vi "Kinesis - MST602 MNA601 - Two Axis Revector.vi"() -> ()   [LabVIEW 2012]
doc: "2D Revector example to centre a NanoTrak tracking power."
uses:
  U:/Kinesis LabVIEW Website Examples/Thorlabs.MotionControl.Controls.dll
  Thorlabs.MotionControl.Controls.dll
  U:/Kinesis LabVIEW Website Examples/Thorlabs.MotionControl.GenericMotorCLI.dll
  Thorlabs.MotionControl.GenericMotorCLI.dll
  U:/Kinesis LabVIEW Website Examples/Thorlabs.MotionControl.ModularRackCLI.dll
  Thorlabs.MotionControl.ModularRackCLI.dll
  U:/Kinesis LabVIEW Website Examples/Thorlabs.MotionControl.GenericNanoTrakCLI.dll
  Thorlabs.MotionControl.GenericNanoTrakCLI.dll
panel:
  out "Step Count":i32
  in  "Move (mm)":sgl=0.01
  in  "?":bool
  in  "?":bool
  in  "Revector Steps":i32=10
  in  "MNA601 SerialNumber":string
  in  "MST602 SerialNumber":string
  in  "ModularStepperControl -   Ch.1":refnum<k24>(container)
  in  "ModularStepperControl - Ch.2":refnum<k24>(container)
  in  "ModularNanoTrakControl":refnum<k24>(container)
  in  "Ch1":u32=4
  in  "Ch2":u32=4
  out "Error":errorcluster
  # "Thorlabs Hardware: \nMST602 Rack Module 2-Ch Stepper Motor Controller \nhttps://www.thorlabs.com/newgrouppage9.cfm?objectgroup_id=1186\n\nMNA601 Rack Module Fiber Auto-alignment Module\nhttps://www.thorlabs.com/newgrouppage9.cfm?objectgroup_id=1187\n\nDescription: The below VI will enable you to connect to a MNA601 & MST602.\nThe MNA601 provides users with an automated fibre alignment facility. It comprises of a PIN photodiode, Transimpedance Amplifier, & a dual channel High Voltage amplifier output circuit for driving two piezo actuators, typically found in our series of high precision flexure stages. The Nanotrak will drive the piezos via a PI servo loop, in a user adjustable circular motion to deduce the signal strength gradient for optimising & automating fibre alignment.\n\nAs the range of the Nanotrak operation is limited to the travel range of the piezo block, a revector routine will check the circle position & the MST602 is employed to control the connected motors, moving the circle position to centre. \n\nAn example of this application setup is pictured whereby the MST602 is driving will drive the internal X & Z piezo blocks of a MAX381 stage. The MAX381 stage is holding an optical fibre aligned to a waveguide in series with secondary receiving fibre via use of Thorlabs flexure stage holder accessories. The secondary fibre is mounted to a secondary co-located MAX302 stage. This fibre is connected to the Optical Input of the MNA601 controller.\n\nThe VI will stop once the revector routine is complete or the user has click 'END'. The user is able to set the number of Revector Iterations (Steps), as well as the step size of the motor movements as well as monitor the current step count.\n\nInstructions: \n1) Connect a MNA601 & MST602 to MMR601 as per the respective product user manuals. These can be connected to any bay in the MMR601 rack.\n2) Enter the module serial numbers below.\n3) Enter the Revector parameters (Move & Revector Iteration Count),\n4) To run the VI, click the run button in the LabVIEW Toolbar.\n5) Once running, the Kinesis UIs will initialise & the VI will wait for you to assign the correct motor types. This can be done by selecting the actuator type on the Kinesis device name on the UI panel & then click 'ACTUATOR SELECTED'\n4) The VI will exit when the revector iteration count is complete or 'END' is clicked."
  # "Notes:"
  # "- Ensure that the appropriate .DLLs are copied into your Project Folder. Check that the correct bit type are used depending on your version of LabVIEW\ni.e. 32-bit or 64-bit.\n\n\n\n\n\n\n\n\n\n\n\n\n\n\n- Open the example VI through the LabVIEW Project Explorer to correctly load the User Interface from Thorlabs.MotionControl.Controls.dll."
  # "Example Image of .NET Controller - VI opened via Project Explorer/ not opened via Project Explorer"
  # "VI Not Opened via Project Explorer"
  # "VI Opened via Project Explorer"
  # "- To explore the range of methods available, please visit the .NET API, included with your Kinesis software.\n\n- For tips on building your own VIs with Thorlabs Motion Control Hardware, please see our LabVIEW Guide here.\nhttps://www.thorlabs.com/newgrouppage9.cfm?objectgroup_id=10285"
  # "Motor Start Position\n(mm)"
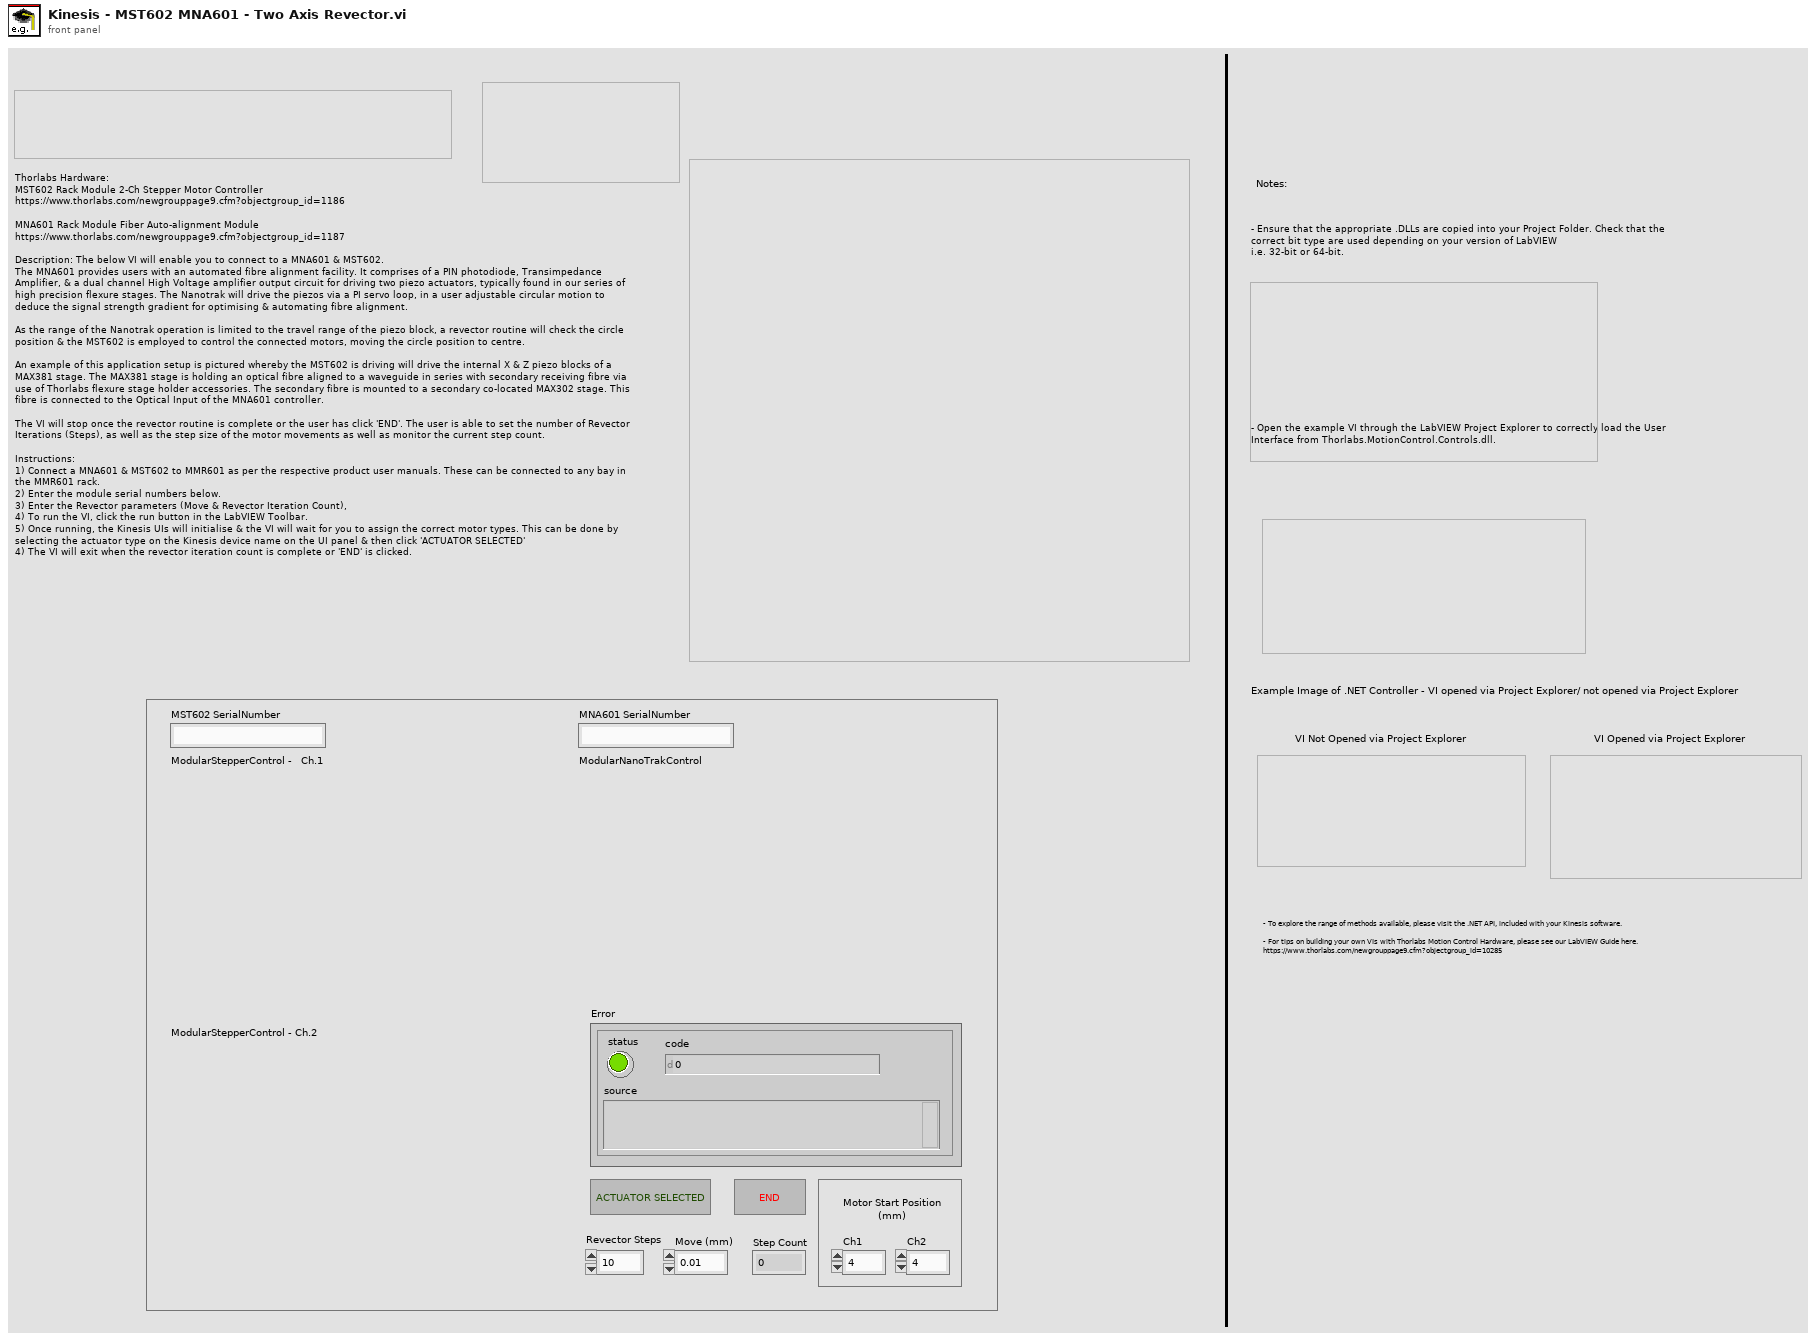
[diagram p1: front panel]
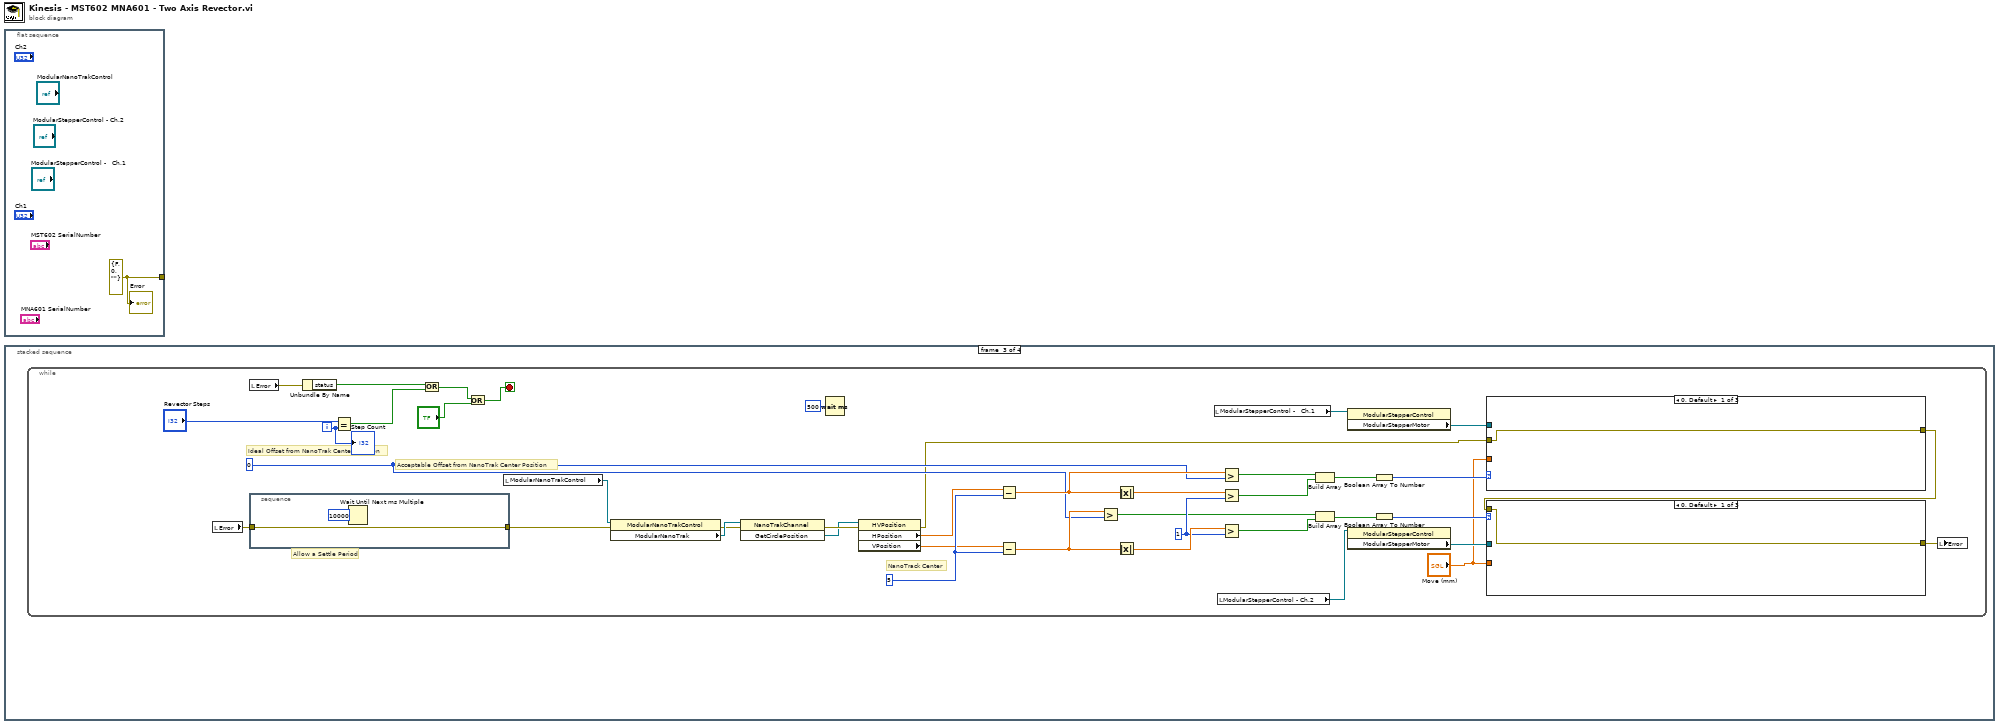
[diagram p0: block diagram]
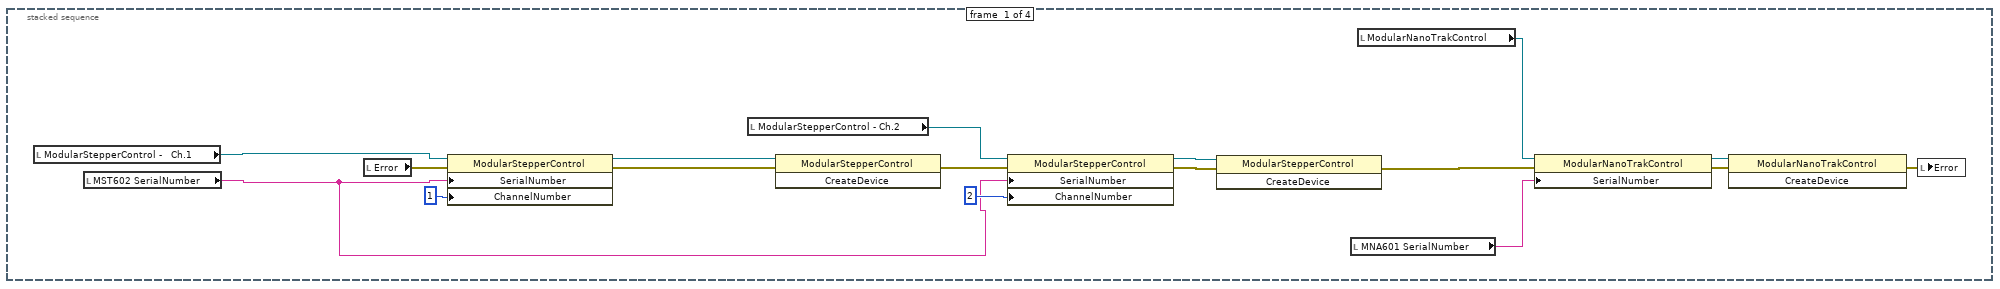
[diagram p2: hidden frame]
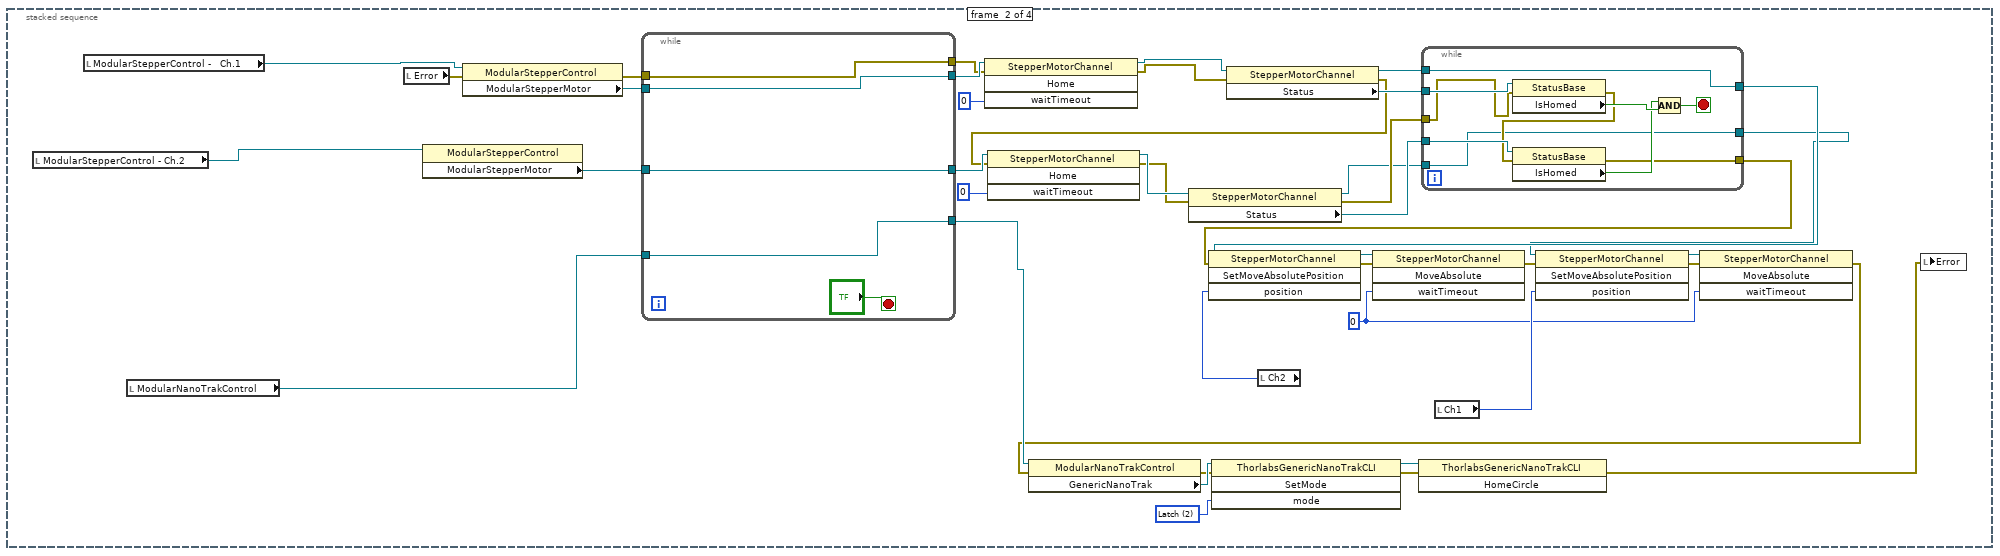
[diagram p3: hidden frame]
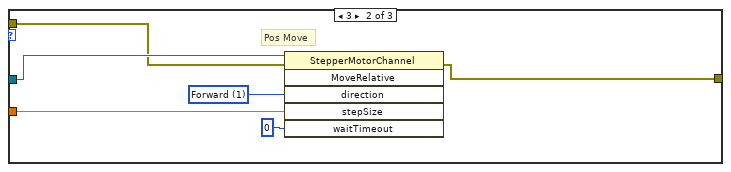
[diagram p4: hidden frame]
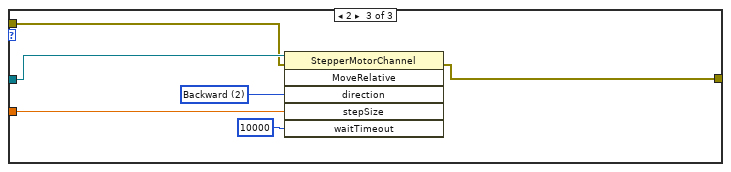
[diagram p5: hidden frame]
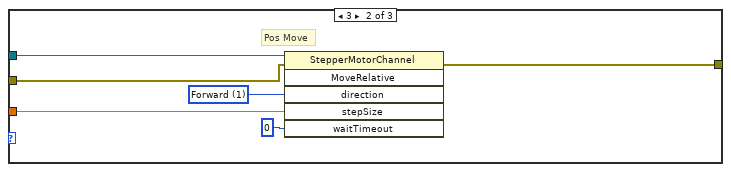
[diagram p6: hidden frame]
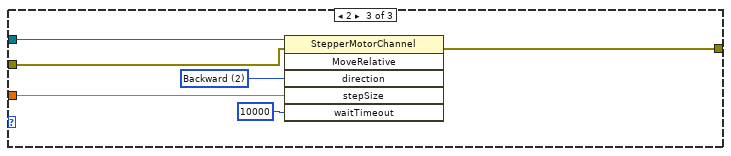
[diagram p7: hidden frame]
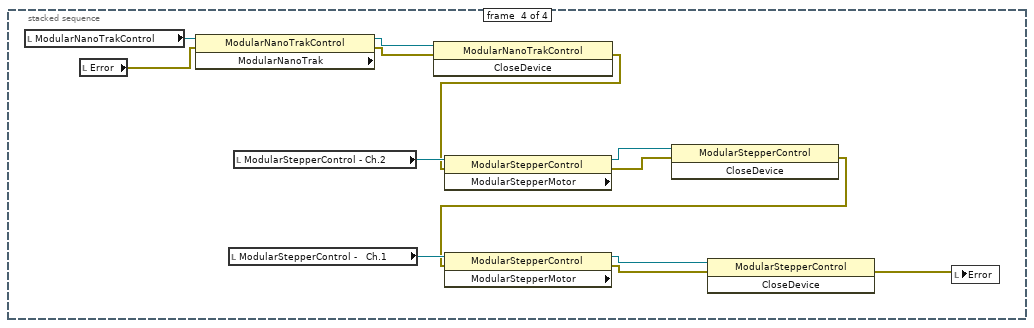
[diagram p8: hidden frame]
diagram:
  n1 = flat-sequence {
    tunnel: [w1] -> _
    frame #0 {
      w1 = errorcluster {"status"=FALSE, "code"=0, "source"=""} ("error in (no error)")
      "Error" <- w1
    }
  }
  n2 = stacked-sequence {
    frame #0 {
      n3 = local read "ModularStepperControl -   Ch.1"() -> (w7:refnum<k24>)
      n4 = local read "MST602 SerialNumber"() -> (w2:string)
      n5 = local read "Error"() -> (w16:errorcluster)
      n6 = property class="ModularStepperControl"(reference=w7, error in=w16, "SerialNumber"=w2, "ChannelNumber"=1) -> (reference out=w18:refnum<k24>, error out=w17:errorcluster)
      n7 = local read "ModularStepperControl - Ch.2"() -> (w3:refnum<k24>)
      n8 = invoke class="ModularStepperControl" method="CreateDevice"(reference=w18, error in=w17) -> (error out=w5:errorcluster)  [unwired: 1 in, 2 out]
      n9 = property class="ModularStepperControl"(reference=w3, error in=w5, "SerialNumber"=w2, "ChannelNumber"=2) -> (reference out=w9:refnum<k24>, error out=w15:errorcluster)
      n10 = invoke class="ModularStepperControl" method="CreateDevice"(reference=w9, error in=w15) -> (error out=w4:errorcluster)  [unwired: 1 in, 2 out]
      n11 = local read "MNA601 SerialNumber"() -> (w12:string)
      n12 = local read "ModularNanoTrakControl"() -> (w13:refnum<k24>)
      n13 = property class="ModularNanoTrakControl"(reference=w13, error in=w4, "SerialNumber"=w12) -> (reference out=w11:refnum<k24>, error out=w10:errorcluster)
      n14 = invoke class="ModularNanoTrakControl" method="CreateDevice"(reference=w11, error in=w10) -> (error out=w8:errorcluster)  [unwired: 1 in, 2 out]
      n15 = local write "Error"(w8) -> ()
    }
    frame #1 {
      w23 = 2 items=["Undefined", "Piezo", "Latch", "Tracking", "HorizontalTracking", "VerticalTracking"] ("mode")
      w48 = 0 ("waitTimeout")
      n16 = local read "ModularStepperControl - Ch.2"() -> (w57:refnum<k24>)
      n17 = local read "ModularStepperControl -   Ch.1"() -> (w58:refnum<k24>)
      n18 = local read "ModularNanoTrakControl"() -> (w21:refnum<k24>)
      n19 = local read "Error"() -> (w56:errorcluster)
      n20 = property class="ModularStepperControl"(reference=w57) -> ("ModularStepperMotor"=w43:refnum<k24>)  [unwired: 1 in, 2 out]
      n21 = property class="ModularStepperControl"(reference=w58, error in=w56) -> (error out=w41:errorcluster, "ModularStepperMotor"=w45:refnum<k24>)  [unwired: 1 out]
      n22 = while {
        tunnel: [w64] -> w46
        tunnel: w45 -> [w64]
        tunnel: [w63] -> w44
        tunnel: w43 -> [w63]
        tunnel: [w62] -> w42
        tunnel: w41 -> [w62]
        tunnel: [w60] -> w22
        tunnel: w21 -> [w60]
        stop <- "?" stop-if-true
      }
      n23 = invoke class="StepperMotorChannel" method="Home"(reference=w46, error in=w42, "waitTimeout"=0) -> (reference out=w37:refnum<k24>, error out=w40:errorcluster)  [unwired: 1 in, 2 out]
      n24 = property class="StepperMotorChannel"(reference=w37, error in=w40) -> (reference out=w30:refnum<k24>, error out=w35:errorcluster, "Status"=w38:refnum<k24>)
      n25 = invoke class="StepperMotorChannel" method="Home"(reference=w44, error in=w35, "waitTimeout"=0) -> (reference out=w36:refnum<k24>, error out=w34:errorcluster)  [unwired: 1 in, 2 out]
      n26 = property class="StepperMotorChannel"(reference=w36, error in=w34) -> (reference out=w28:refnum<k24>, error out=w33:errorcluster, "Status"=w39:refnum<k24>)
      n27 = local read "Ch2"() -> (w54:u32)
      n28 = while {
        tunnel: w39 -> [w71]
        tunnel: w38 -> [w70]
        tunnel: w33 -> [w68]
        tunnel: [w67] -> w32
        tunnel: [w66] -> w31
        tunnel: w30 -> [w66]
        tunnel: [w65] -> w29
        tunnel: w28 -> [w65]
        stop <- w72 stop-if-true
        n29 = property class="StatusBase"(reference=w70, error in=w68) -> (error out=w69:errorcluster, "IsHomed"=w74:bool)  [unwired: 1 out]
        n30 = property class="StatusBase"(reference=w71, error in=w69) -> (error out=w67:errorcluster, "IsHomed"=w73:bool)  [unwired: 1 out]
        n31 = Compound Arithmetic op=AND(w73, w74) -> (w72:bool)
      }
      n32 = invoke class="StepperMotorChannel" method="SetMoveAbsolutePosition"(reference=w31, error in=w32, "position"=w54) -> (reference out=w51:refnum<k24>, error out=w50:errorcluster)  [unwired: 1 in, 2 out]
      n33 = invoke class="StepperMotorChannel" method="MoveAbsolute"(reference=w51, error in=w50, "waitTimeout"=w48) -> (error out=w55:errorcluster)  [unwired: 1 in, 3 out]
      n34 = local read "Ch1"() -> (w53:u32)
      n35 = invoke class="StepperMotorChannel" method="SetMoveAbsolutePosition"(reference=w29, error in=w55, "position"=w53) -> (reference out=w52:refnum<k24>, error out=w49:errorcluster)  [unwired: 1 in, 2 out]
      n36 = invoke class="StepperMotorChannel" method="MoveAbsolute"(reference=w52, error in=w49, "waitTimeout"=w48) -> (error out=w20:errorcluster)  [unwired: 1 in, 3 out]
      n37 = property class="ModularNanoTrakControl"(reference=w22, error in=w20) -> (error out=w25:errorcluster, "GenericNanoTrak"=w27:refnum<k24>)  [unwired: 1 out]
      n38 = invoke class="ThorlabsGenericNanoTrakCLI" method="SetMode"(reference=w27, error in=w25, "mode"=w23) -> (reference out=w26:refnum<k24>, error out=w24:errorcluster)  [unwired: 1 in, 2 out]
      n39 = invoke class="ThorlabsGenericNanoTrakCLI" method="HomeCircle"(reference=w26, error in=w24) -> (error out=w19:errorcluster)  [unwired: 1 in, 2 out]
      n40 = local write "Error"(w19) -> ()
    }
    frame #2 {
      n41 = while {
        i -> [w101]
        stop <- w80 stop-if-true
        w109 = 0
        w111 = 1
        w115 = 5
        # "Allow a Settle Period"
        # "Acceptable Offset from NanoTrak Center Position"
        # "Ideal Offset from NanoTrak Center Position"
        # "NanoTrack Center"
        n42 = local read "Error"() -> (w98:errorcluster)
        n43 = local read "Error"() -> (w87:errorcluster)
        n44 = stacked-sequence {
          tunnel: w98 -> [w130]
          tunnel: [w130] -> w92
          frame #0 {
            n45 = Wait Until Next ms Multiple(millisecond multiple=10000) -> ()  [unwired: 1 out]
          }
        }
        n46 = Unbundle By Name(w87) -> ("status"=w100:bool)
        n47 = Equal?(x="Revector Steps", y=w101) -> (x = y?=w99:bool)
        n48 = Or(x=w100, y=w99) -> (x .or. y?=w81:bool)
        n49 = Or(x=w81, y="?") -> (x .or. y?=w80:bool)
        n50 = local read "ModularNanoTrakControl"() -> (w97:refnum<k24>)
        n51 = property class="ModularNanoTrakControl"(reference=w97, error in=w92) -> (error out=w91:errorcluster, "ModularNanoTrak"=w96:refnum<k24>)  [unwired: 1 out]
        n52 = invoke class="NanoTrakChannel" method="GetCirclePosition"(reference=w96, error in=w91) -> (error out=w95:errorcluster, "GetCirclePosition"=w86:refnum<k24>)  [unwired: 1 in, 1 out]
        n53 = Wait (ms)(milliseconds to wait=u32 500) -> ()  [unwired: 1 out]
        n54 = property class="HVPosition"(reference=w86, error in=w95) -> (error out=w78:errorcluster, "HPosition"=w94:dbl, "VPosition"=w93:dbl)  [unwired: 1 out]
        n55 = Subtract(x=w94, y=w115) -> (x-y=w113:dbl)
        n56 = Subtract(x=w93, y=w115) -> (x-y=w110:dbl)
        n57 = Greater?(x=w110, y=w109) -> (0:w106:bool)
        n58 = Absolute Value(x=w113) -> (abs(x)=w114:dbl)
        n59 = Absolute Value(x=w110) -> (abs(x)=w112:dbl)
        n60 = local read "ModularStepperControl -   Ch.1"() -> (w90:refnum<k24>)
        n61 = local read "ModularStepperControl - Ch.2"() -> (w88:refnum<k24>)
        n62 = Greater?(x=w113, y=w109) -> (0:w108:bool)
        n63 = Greater?(x=w114, y=w111) -> (0:w107:bool)
        n64 = Greater?(x=w112, y=w111) -> (0:w105:bool)
        n65 = Build Array(w108, w107) -> (w104:bool[])
        n66 = Build Array(w106, w105) -> (w103:bool[])
        n67 = property class="ModularStepperControl"(reference=w90) -> ("ModularStepperMotor"=w84:refnum<k24>)  [unwired: 1 in, 2 out]
        n68 = property class="ModularStepperControl"(reference=w88) -> ("ModularStepperMotor"=w85:refnum<k24>)  [unwired: 1 in, 2 out]
        n69 = Boolean Array To Number(Boolean array=w104) -> (number=w102:u32)
        n70 = Boolean Array To Number(Boolean array=w103) -> (number=w89:u32)
        n71 = case shown="0, Default" w102 {
          tunnel: "Move (mm)" -> [_ w135 w140]
          tunnel: w84 -> [_ w137 w141]
          tunnel: w78 -> [w131 w133 w139]
          tunnel: [w131 w132 w138] -> w77
          frame 0, Default {
          }
          frame 3 {
            w136 = 1 items=["Forward"=1, "Backward"=2] ("direction")
            # "Pos Move"
            n72 = invoke class="StepperMotorChannel" method="MoveRelative"(reference=w137, error in=w133, "direction"=w136, "stepSize"=w135, "waitTimeout"=0) -> (error out=w132:errorcluster)  [unwired: 1 in, 5 out]
          }
          frame 2 {
            w143 = 2 items=["Forward"=1, "Backward"=2] ("direction")
            n73 = invoke class="StepperMotorChannel" method="MoveRelative"(reference=w141, error in=w139, "direction"=w143, "stepSize"=w140, "waitTimeout"=10000) -> (error out=w138:errorcluster)  [unwired: 1 in, 5 out]
          }
        }
        n74 = case shown="0, Default" w89 {
          tunnel: "Move (mm)" -> [_ w120 w125]
          tunnel: w85 -> [_ w122 w126]
          tunnel: w77 -> [w116 w118 w124]
          tunnel: [w116 w117 w123] -> w76
          frame 0, Default {
          }
          frame 3 {
            w121 = 1 items=["Forward"=1, "Backward"=2] ("direction")
            # "Pos Move"
            n75 = invoke class="StepperMotorChannel" method="MoveRelative"(reference=w122, error in=w118, "direction"=w121, "stepSize"=w120, "waitTimeout"=0) -> (error out=w117:errorcluster)  [unwired: 1 in, 5 out]
          }
          frame 2 {
            w128 = 2 items=["Forward"=1, "Backward"=2] ("direction")
            n76 = invoke class="StepperMotorChannel" method="MoveRelative"(reference=w126, error in=w124, "direction"=w128, "stepSize"=w125, "waitTimeout"=10000) -> (error out=w123:errorcluster)  [unwired: 1 in, 5 out]
          }
        }
        n77 = local write "Error"(w76) -> ()
        "Step Count" <- w101
      }
    }
    frame #3 {
      n78 = local read "ModularNanoTrakControl"() -> (w155:refnum<k24>)
      n79 = local read "Error"() -> (w144:errorcluster)
      n80 = property class="ModularNanoTrakControl" props=["ModularNanoTrak"](reference=w155, error in=w144) -> (reference out=w151:refnum<k24>, error out=w150:errorcluster)  [unwired: 1 out]
      n81 = local read "ModularStepperControl -   Ch.1"() -> (w156:refnum<k24>)
      n82 = local read "ModularStepperControl - Ch.2"() -> (w154:refnum<k24>)
      n83 = invoke class="ModularNanoTrakControl" method="CloseDevice"(reference=w151, error in=w150) -> (error out=w149:errorcluster)  [unwired: 1 in, 2 out]
      n84 = property class="ModularStepperControl" props=["ModularStepperMotor"](reference=w154, error in=w149) -> (reference out=w153:refnum<k24>, error out=w148:errorcluster)  [unwired: 1 out]
      n85 = invoke class="ModularStepperControl" method="CloseDevice"(reference=w153, error in=w148) -> (error out=w147:errorcluster)  [unwired: 1 in, 2 out]
      n86 = property class="ModularStepperControl" props=["ModularStepperMotor"](reference=w156, error in=w147) -> (reference out=w152:refnum<k24>, error out=w146:errorcluster)  [unwired: 1 out]
      n87 = invoke class="ModularStepperControl" method="CloseDevice"(reference=w152, error in=w146) -> (error out=w145:errorcluster)  [unwired: 1 in, 2 out]
      n88 = local write "Error"(w145) -> ()
    }
  }
